vi "WinCI Is File In Local Path.vi"(8 "error in (no error)":errorcluster, 10 "files":path[](array[path]), 11 "source control reference in":T1) -> (0 "error out":errorcluster, 2 "in local path?":bool[](array[boolean]), 3 "source control reference out":T1)   [LabVIEW 2017, in "NI_SCC_WinCI.lvlib"]
uses:
  <vilib>/SourceControl/Providers/WinCI/NI_SCC_WinCI.lvlib
  <vilib>/SourceControl/sccapi/SCCAPI Refnum.ctl
  <vilib>/SourceControl/sccapi/NI_SCC.lvlib
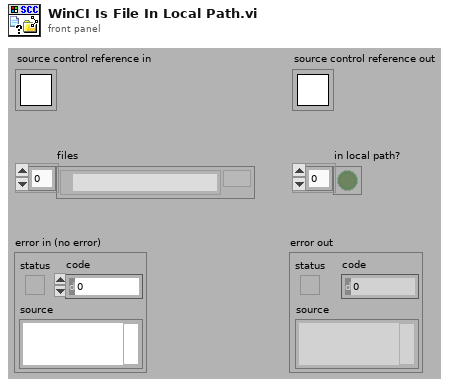
[diagram p1: front panel]
types:
  T1 = typedef "NI_SCC.lvlib/SCCAPI Refnum.ctl" = refnum<k1>
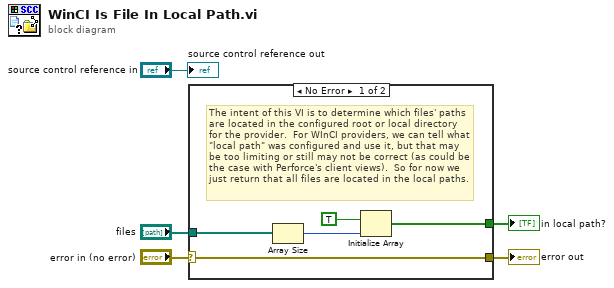
[diagram p0: block diagram]
diagram:
  n1 = case shown="No Error" "error in (no error)" {
    selector: "error in (no error)" -> [w8 w11]
    tunnel: [w8 w11] -> w4
    tunnel: "files" -> [w10 _]
    tunnel: [w9 _] -> w2
    frame No Error {
      # "The intent of this VI is to determine which files' paths are located in the configured root or local directory for the provider.  For WInCI providers, we can tell what \"local path\" was configured and use it, but that may be too limiting or still may not be correct (as could be the case with Perforce's client views).  So for now we just return that all files are located in the local paths."
      n2 = Array Size(array=w10) -> (size(s)=w7:i32)
      n3 = Initialize Array(TRUE, w7) -> (w9:bool[])
    }
    frame Error {
    }
  }
  "error out" <- w4
  "in local path?" <- w2
  "source control reference out" <- "source control reference in"
